vi "Find (single).vi"(8 "error in (no error)":errorcluster, 10 "Key":string, 11 "Parameter to Hardware Map in":refnum<class "Parameter to Hardware Map.lvclass">) -> (0 "error out":errorcluster, 1 "Found?":bool, 2 "Key-Value Pair":T1, 3 "Parameter to Hardware Map out":refnum<class "Parameter to Hardware Map.lvclass">)   [LabVIEW 2020, in "Parameter to Hardware Map.lvclass"]
doc: "Find the element from the map matching the given key."
uses:
  Parameter to Hardware Map.lvclass
  Controller/Generic Plugin.lvclass
  Pair.ctl
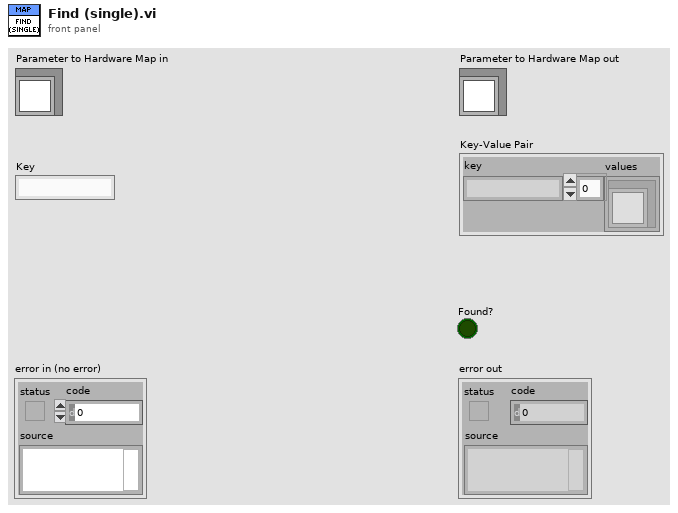
[diagram p1: front panel]
types:
  T1 = typedef "Parameter to Hardware Map.lvclass/Pair.ctl" = cluster{"key":string, "values":refnum<class "Generic Plugin.lvclass">[]}
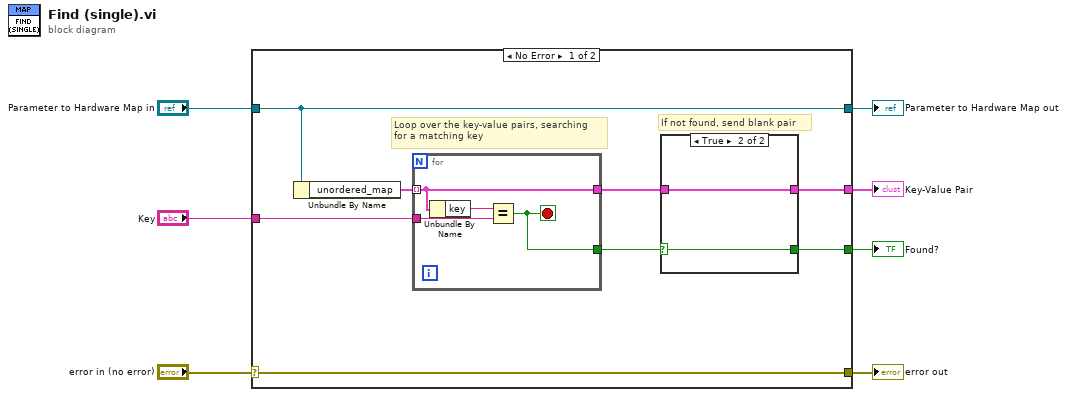
[diagram p0: block diagram]
diagram:
  n1 = case shown="No Error" "error in (no error)" {
    selector: "error in (no error)" -> [w15 w24]
    tunnel: [w15 w24] -> w6
    tunnel: [w14 w23] -> w4
    tunnel: "Parameter to Hardware Map in" -> [w14 w23]
    tunnel: "Key" -> [w12 _]
    tunnel: [w11 _] -> w1
    tunnel: [w9 _] -> w2
    frame No Error {
      # "If not found, send blank pair"
      # "Loop over the key-value pairs, searching\nfor a matching key"
      n2 = Unbundle By Name(w14) -> ("unordered_map"=w13:T1[])
      n3 = for {
        tunnel: w13 -> [w20] mode=indexing
        tunnel: w12 -> [w21]
        tunnel: [w20] -> w8
        tunnel: [w19] -> w10
        stop <- w19 stop-if-true
        n4 = Unbundle By Name(w20) -> ("key"=w22:string)
        n5 = Equal?(x=w22, y=w21) -> (x = y?=w19:bool)
      }
      n6 = case shown="True" w10 {
        selector: w10 -> [w16 w18]
        tunnel: [_ w17] -> w11
        tunnel: [w16 w18] -> w9
        tunnel: w8 -> [_ w17]
        frame False {
        }
        frame True {
        }
      }
    }
    frame Error {
    }
  }
  "error out" <- w6
  "Parameter to Hardware Map out" <- w4
  "Found?" <- w2
  "Key-Value Pair" <- w1
